vi "str2Float.vi"(0 "string":string) -> (1 "is a floating":bool, 2 "number":dbl format="%.2f")   [LabVIEW 2014]
doc: "Returns an DBL corresponding to the floating value of the input string.\nIf the string does not represent just a float number, the VI returns 0.0 and FALSE."
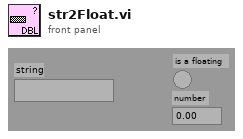
[diagram p1: front panel]
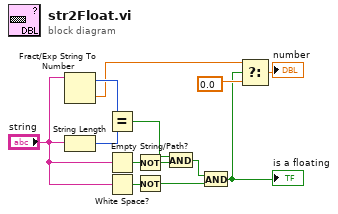
[diagram p0: block diagram]
diagram:
  n1 = Fract/Exp String To Number(string="string") -> (offset past number=w10:i32, number=w9:dbl)  [unwired: 3 in]
  n2 = String Length(string="string") -> (length=w13:i32)
  n3 = Equal?(x=w10, y=w13) -> (x = y?=w2:bool)
  n4 = Empty String/Path?(string/path="string") -> (empty?=w8:bool)
  n5 = White Space?(1:"string") -> (0:w6:bool)
  n6 = Not(x=w8) -> (.not. x?=w7:bool)
  n7 = Not(x=w6) -> (.not. x?=w3:bool)
  n8 = And(x=w2, y=w7) -> (x .and. y?=w4:bool)
  n9 = And(x=w4, y=w3) -> (x .and. y?=w1:bool)
  "is a floating" <- w1
  n10 = Select(t=w9, s=w1, f=0.0) -> (s? t:f=→"number":dbl)
